vi "Overriding Diode D1.vi"(8 "error in":errorcluster) -> (0 "error out":errorcluster, 1 "PASS/FAIL":bool, 3 "VHeatFuse_noload":string)   [LabVIEW 2009]
uses:
  Digit IO PCI 6503/Digit IO control.ctl
  Global/Global 1.vi
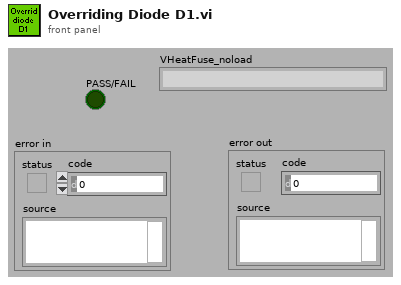
[diagram p1: front panel]
types:
  T1 = typedef "Digit IO control.ctl" = enum16{"Pull X1_4 Low", "Disconnect Pull X1_4 Low", "Down Cylinder", "Disconnect Down Cylinder", "Load X1_1_5", "Disconnect Load X1_1_5", "Measu X1_1_5", "Disconnect Measu X1_1_5", "Measu Z1_1_5", "Disconnect Measu Z1_1_5", "Power X1_1", "Disconnect Power X1_1", "RS232 Power", "Disconnect RS232 Power", "Card Cylinder", "Disconnect Card Cylinder", "Fail LED", "Disconnect Fail LED", "LCA Power", "Disconnect LCA Power", "BeyondCylinderDowndigit", "Disconnect BeyondCylinderDowendigit", "Frequency", "Disconnect Frequency", "Measu Current", "Disconnect Measu Current", "Measu current_1", "Disconnect Measu current_1", "Digit ALL", "Disconnect Digit ALL", "PASS LED", "Disconnect PASS LED", "Load Z1_1_3", "Disconnect Load Z1_1_3", "RS232 Connect", "Disconnect RS232 Connect", "Power Z1_7", "Disconnect Power Z1_7", "Pull Z_1_5  low", "Disconnect Pull Z_1_5  low", "Connect LCA_1", "Disconnect LCA_1", "short LCA", "Disconnect short LCA", "PT100", "Disconnect PT100", "NO connect", "Disconnect NO connect"}
  T2 = cluster{"VHEATFUSENOLOADMIN":string, "VHEATFUSELOADMAX":string, "VOVERRIDEDIODEMIN":string, "TDIFFMAX":string, "MEASFREQMAX":string, "MEASFREQMIN":string, "VOVER":string, "VMIDDLE":string, "VUNDER":string, "VNORESET":string, "VRESET":string, "WAITPING":string, "LRFID":string, "RFIDUID":string, "EXTEESIZE":string, "LCUTYPE":string, "LCUSUBTYPE":string, "TEVN":string, "BOOTVER":string, "APPVER":string, "ISLEEPMAX":string, "TSLEEP":string, "APPWAIT":string, "DBWAIT":string}
  T3 = cluster{"People":string, "product  number":string, "Test time":string, "VHeatFuse_noload":string, "VHeatFuse_load":string, "VoverrideDiode":string, "Test firmware upload via X1":string, "TemperAddress":string, "Troom":string, "TLCU":string, "Adjustment factor":string, "MeasuredFreq":string, "I2C communication":string, "Light-emitting diode on Z2":string, "Battery warning/inhibit":string, "Reset by IC10":string, "External EEPROM":string, "RFID card detection and reading RFID":string, "Production parameters in internal EEPROM":string, "Current consumption in sleep mode":string, "Application and database upload":string, "Test result":string, "Table head[22]":string, "Table head[23]":string}
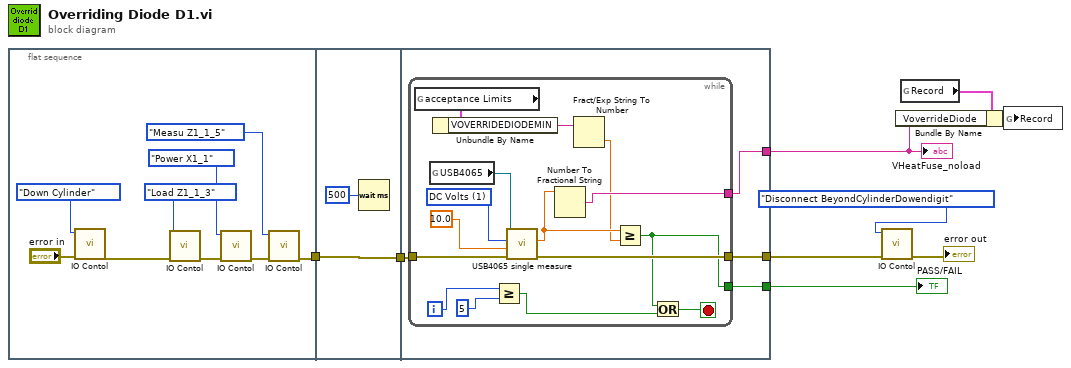
[diagram p0: block diagram]
diagram:
  n1 = flat-sequence {
    tunnel: [w17] -> w2
    tunnel: w2 -> [w20]
    tunnel: [w20] -> w6
    tunnel: w6 -> [w24]
    tunnel: [w23] -> w3
    tunnel: [w22] -> w1
    tunnel: [w21] -> w7
    frame #0 {
      n2 = call "IO Contol.vi"("error in"="error in", "IO Operation"=Digit_IO_control."Down Cylinder" ("Enum")) -> ("error out"=w10:errorcluster)  [unwired: 9 out]
      n3 = call "IO Contol.vi"("error in"=w10, "IO Operation"=Digit_IO_control."Load Z1_1_3" ("Enum")) -> ("error out"=w16:errorcluster)  [unwired: 9 out]
      n4 = call "IO Contol.vi"("error in"=w16, "IO Operation"=Digit_IO_control."Power X1_1" ("Enum")) -> ("error out"=w18:errorcluster)  [unwired: 9 out]
      n5 = call "IO Contol.vi"("error in"=w18, "IO Operation"=Digit_IO_control."Measu Z1_1_5" ("Enum")) -> ("error out"=w17:errorcluster)  [unwired: 9 out]
    }
    frame #1 {
      n6 = Wait (ms)(milliseconds to wait=u32 500) -> ()  [unwired: 1 out]
    }
    frame #2 {
      n7 = while {
        tunnel: w24 -> [w37]
        tunnel: [w32] -> w22
        tunnel: [w29] -> w23
        tunnel: [w28] -> w21
        i -> [w35]
        stop <- w36 stop-if-true
        w39 = 1 items=["DC Volts"=1, "AC Volts"=2, "DC Current"=3, "AC Current"=4, "2-Wire Resistance"=5, "4-Wire Resistance"=101, "Frequency"=104, "Period"=105, "AC Volts DC Coupled"=1001, "Diode"=1002, "Waveform Voltage"=1003, "Waveform Current"=1004, "Capacitance"=1005, "Inductance"=1006, "Temperature"=108] ("Configuration:Function")
        n8 = global read "Global 1.vi" "acceptance Limits"() -> (w27:T2)
        n9 = global read "Global 1.vi" "USB4065"() -> (w31:refnum<k15>)
        n10 = Unbundle By Name(w27) -> ("VOVERRIDEDIODEMIN"=w26:string)
        n11 = Greater Or Equal?(x=w35, y=5) -> (x >= y?=w33:bool)
        n12 = call "USB4065 single measure.vi"("error in (no error)"=w37, "Configuration:Range"=10.0, "Configuration:Function"=w39, "Instrument Descriptor"=w31) -> ("error out"=w32:errorcluster, "Measurement"=w30:dbl)  [unwired: 6 out]
        n13 = Number To Fractional String(number=w30) -> (F-format string=w29:string)  [unwired: 3 out]
        n14 = Fract/Exp String To Number(string=w26) -> (number=w25:dbl)  [unwired: 4 out]
        n15 = Greater Or Equal?(x=w30, y=w25) -> (x >= y?=w28:bool)
        n16 = Or(x=w28, y=w33) -> (x .or. y?=w36:bool)
      }
    }
  }
  n17 = call "IO Contol.vi"("error in"=w1, "IO Operation"=Digit_IO_control."Disconnect BeyondCylinderDowendigit" ("Enum")) -> ("error out"=→"error out":errorcluster)  [unwired: 9 out]
  n18 = global read "Global 1.vi" "Record"() -> (w5:T3)
  n19 = Bundle By Name(cluster=w5, "VoverrideDiode"=w3) -> (w4:T3)
  n20 = global write "Global 1.vi" "Record"(w4) -> ()
  "VHeatFuse_noload" <- w3
  "PASS/FAIL" <- w7
